vi "DB Tools Parser.vi"(3 "error in (no error)":errorcluster, 4 "flatten cluster? (F)":bool, 5 "variant":variant) -> (0 "error out":errorcluster, 2 "parameters":T1[](array[typedef]))   [LabVIEW 2017, in "NI_Database_API.lvlib"]
doc: "This VI converts any type of data as specified by the variant input into an array of clusters of data parameters used by databases. The parameters include the data name, data type, data direction (input, output, etc.), and the data value. If the variant input is a cluster the parameters array will contain an element for each element of the cluster. You can also specify to flatten the cluster to create a single parameter of binary data type."
uses:
  <vilib>/addons/database/NI_Database_API.lvlib
  <vilib>/addons/database/Auxilliary.llb/DB Tools Parameter Info.ctl
  <vilib>/addons/database/Auxilliary.llb/DB Tools DataTypes.ctl
  <vilib>/addons/database/Auxilliary.llb/DB Tools Parameter Dir.ctl
  <vilib>/Utility/VariantDataType/Type.ctl
  <vilib>/Utility/VariantDataType/VariantType.lvlib
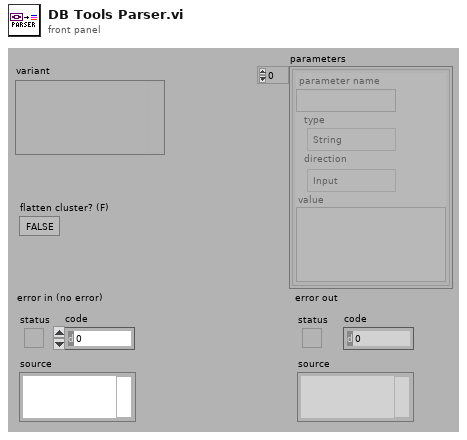
[diagram p1: front panel]
types:
  T1 = typedef "NI_Database_API.lvlib/DB Tools Parameter Info.ctl" = cluster{"parameter name":string, "type":T2, "direction":T3, "value":variant}
  T2 = typedef "NI_Database_API.lvlib/DB Tools DataTypes.ctl" = enum16{"String", "Long (I32)", "Single (SGL)", "Double (DBL)", "Date/Time", "Binary"}
  T3 = typedef "NI_Database_API.lvlib/DB Tools Parameter Dir.ctl" = enum32{"Input", "Output", "Input/Output", "Return Value"}
  T4 = typedef "Database Connectivity Toolkit.lvlib/DB Tools LV Type.ctl" = enum16{"Unsupported", "Boolean", "I8", "I16", "I32", "U8", "U16", "U32", "SGL", "DBL", "EXT", "CSG", "CDB", "CXT", "String", "Path", "Picture", "I/O Channel", "Array", "Cluster", "Variant", "WDT"}
  T5 = typedef "VariantType.lvlib/Type.ctl" = enum8{"Invalid Type", "Void", "I8", "I16", "I32", "I64", "U8", "U16", "U32", "U64", "Single Float", "Double Float", "Extended Float", "Single Complex", "Double Complex", "Extended Complex", "Enum U8", "Enum U16", "Enum U32", "Enum U64", "Single Float With Unit", "Double Float With Unit", "Extended Float With Unit", "Single Complex with Unit", "Double Complex with Unit", "Extended Complex with Unit", "Boolean", "String", "Path", "Picture", "Tag", "Array", "Cluster", "Variant", "LV Variant", "Waveform", "Timestamp", "Digital Waveform", "Digital Data", "ExpressData", "Refnum", "External Data", "VI", "Poly VI", "LabVIEW Class Instance", "Fixed Point"}
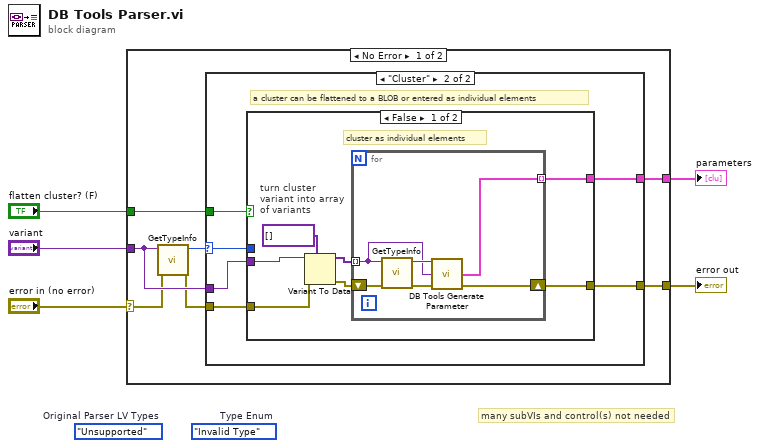
[diagram p0: block diagram]
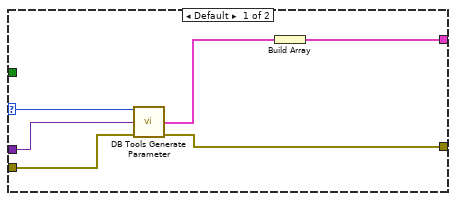
[diagram p2: hidden frame]
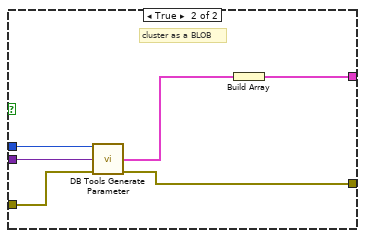
[diagram p3: hidden frame]
diagram:
  (unwired) DB_Tools_LV_Type."Unsupported"  # Original Parser LV Types
  (unwired) Type."Invalid Type"  # Type Enum
  # "many subVIs and control(s) not needed"
  n1 = case shown="No Error" "error in (no error)" {
    selector: "error in (no error)" -> [w7 w44]
    tunnel: [w12 w44] -> w4
    tunnel: "variant" -> [w10 _]
    tunnel: [w9 _] -> w2
    tunnel: "flatten cluster? (F)" -> [w8 _]
    frame No Error {
      n2 = call <vilib>:"GetTypeInfo.vi"("error in (no error)"=w7, "Variant"=w10) -> ("error out"=w6:errorcluster, "Type Enum"=w11:T5)  [unwired: 5 in, 3 out]
      n3 = case shown="\"Cluster\"" w11 {
        selector: w11 -> [w18 w19]
        tunnel: [w15 w21] -> w12
        tunnel: [w13 w23] -> w9
        tunnel: w6 -> [w16 w22]
        tunnel: w10 -> [w17 w20]
        tunnel: w8 -> [_ w24]
        frame Default {
          n4 = call <vilib>:"DB Tools Generate Parameter.vi"("Type Enum"=w18, "Variant data"=w17, "error in (no error)"=w16) -> ("parameter information"=w14:T1, "error out"=w15:errorcluster)  [unwired: 11 in]
          n5 = Build Array(w14) -> (w13:T1[])
        }
        frame "Cluster" {
          # "a cluster can be flattened to a BLOB or entered as individual elements"
          n6 = case shown="False" w24 {
            tunnel: [w25 w40] -> w23
            tunnel: w22 -> [w28 w39]
            tunnel: [w26 w38] -> w21
            tunnel: w20 -> [w31 w42]
            tunnel: w19 -> [_ w43]
            frame False {
              # "cluster as individual elements"
              # "turn cluster variant into array of variants"
              n7 = Variant To Data(error in=w28, type=variant[] [], Variant=w31) -> (data=w29:variant[], error out=w27:errorcluster)
              n8 = for {
                tunnel: w29 -> [w34] mode=indexing
                shift-right: [w33] -> w26
                shift-left: w27 -> [w35]
                tunnel: [w32] -> w25 mode=indexing
                n9 = call <vilib>:"GetTypeInfo.vi"("error in (no error)"=w35, "Variant"=w34) -> ("error out"=w36:errorcluster, "Type Enum"=w37:T5)  [unwired: 5 in, 3 out]
                n10 = call <vilib>:"DB Tools Generate Parameter.vi"("Type Enum"=w37, "Variant data"=w34, "error in (no error)"=w36) -> ("parameter information"=w32:T1, "error out"=w33:errorcluster)  [unwired: 11 in]
              }
            }
            frame True {
              # "cluster as a BLOB"
              n11 = call <vilib>:"DB Tools Generate Parameter.vi"("Type Enum"=w43, "Variant data"=w42, "error in (no error)"=w39) -> ("parameter information"=w41:T1, "error out"=w38:errorcluster)  [unwired: 11 in]
              n12 = Build Array(w41) -> (w40:T1[])
            }
          }
        }
      }
    }
    frame Error {
    }
  }
  "error out" <- w4
  "parameters" <- w2
